vi "Get Name.vi"(1 "ID":u16) -> (0 "Name":string)   [LabVIEW 2018]
panel:
  out "subarray":string[](array[string])
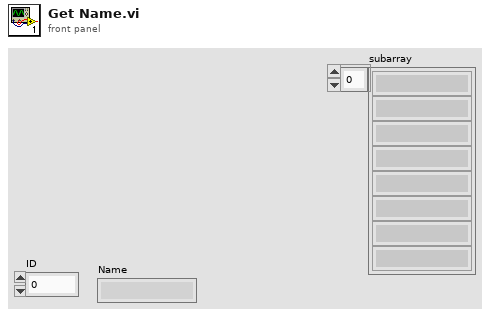
[diagram p1: front panel]
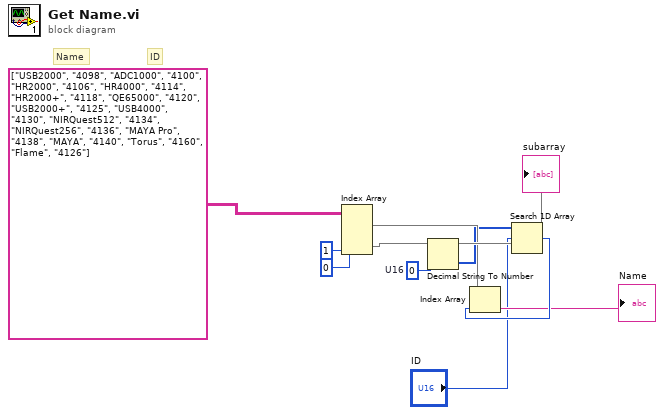
[diagram p0: block diagram]
diagram:
  w8 = u16 0  # U16
  # "ID"
  # "Name"
  n1 = Index Array(array=string[][] [["USB2000", "4098"], ["ADC1000", "4100"], ["HR2000", "4106"], ["HR4000", "4114"], ["HR2000+", "4118"], ["QE65000", "4120"], ["USB2000+", "4125"], ["USB4000", "4130"], ["NIRQuest512", "4134"], ["NIRQuest256", "4136"], ["MAYA Pro", "4138"], ["MAYA", "4140"], ["Torus", "4160"], ["Flame", "4126"]] ("Ocean Optics Definitions"), index (col) #1=0 ("disabled index (col)"), index (col) #2=1 ("disabled index (col)")) -> (element #1=w7:string[], element #2=w9:string[])  [unwired: 2 in]
  "subarray" <- w9
  n2 = Decimal String To Number(string=w9, default (0L)=w8) -> (number=w6:u16[])  [unwired: 1 in, 1 out]
  n3 = Search 1D Array(1D array=w6, element="ID") -> (index of element=w5:i32)  [unwired: 1 in]
  n4 = Index Array(array=w7, index=w5) -> (element=→"Name":string)
